vi "自我介绍.vi"(8 "error in (no error)":errorcluster caption="错误输入（无错误）", 11 "鸭子库.lvlib:绿头鸭.lvclass":refnum<class "绿头鸭.lvclass">) -> (0 "error out":errorcluster caption="错误输出", 3 "鸭子库.lvlib:绿头鸭.lvclass":refnum<class "绿头鸭.lvclass">)   [LabVIEW 2022 SP3, in "鸭子库.lvlib" / "绿头鸭.lvclass"]
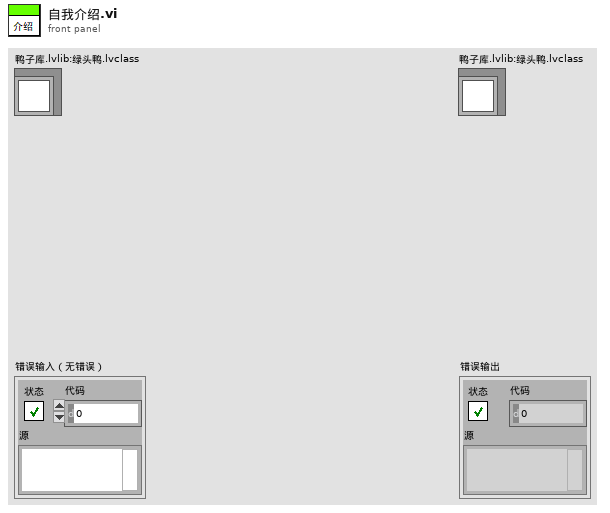
[diagram p1: front panel]
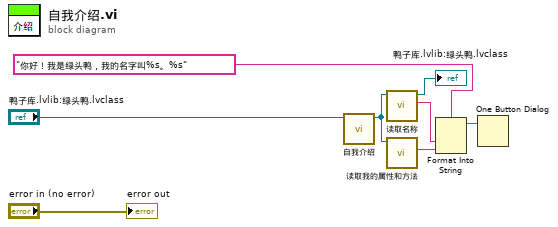
[diagram p0: block diagram]
diagram:
  n1 = call-parent "自我介绍.vi"("鸭子 输入"="鸭子库.lvlib:绿头鸭.lvclass") -> ("鸭子 输出"=w1:refnum<class "绿头鸭.lvclass">)  [unwired: 9 in, 1 out]
  n2 = call "读取名称.vi"("鸭子库.lvlib:鸭子.lvclass"=w1) -> ("名称"=w4:string, "鸭子库.lvlib:鸭子.lvclass"=→"鸭子库.lvlib:绿头鸭.lvclass":refnum<class "绿头鸭.lvclass">)  [unwired: 8 in, 1 out]
  n3 = call "读取我的属性和方法.vi"("鸭子输入"=w1) -> ("我的属性和方法"=w5:string)  [unwired: 8 in, 2 out]
  n4 = Format Into String(format string="你好！我是绿头鸭，我的名字叫%s。%s" ("格式字符串"), w4, w5) -> (resulting string=w6:string)  [unwired: 2 in, 1 out]
  n5 = One Button Dialog(message=w6) -> ()  [unwired: 1 in, 1 out]
  "error out" <- "error in (no error)"
